vi "String_Time_fill_if_one_digit.vi"(11 "String":string) -> (3 "String 2":string)   [LabVIEW 2018]
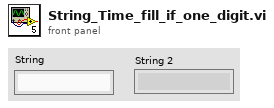
[diagram p1: front panel]
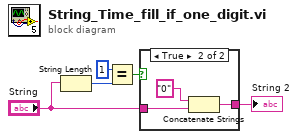
[diagram p0: block diagram]
diagram:
  n1 = String Length(string="String") -> (length=w5:i32)
  n2 = Equal?(x=1, y=w5) -> (x = y?=w3:bool)
  n3 = case shown="True" w3 {
    tunnel: "String" -> [w6 w9]
    tunnel: [w6 w7] -> w1
    frame False {
    }
    frame True {
      n4 = Concatenate Strings("0", w9) -> (w7:string)
    }
  }
  "String 2" <- w1
